vi "ROI entry-Previous ROI compat.vi"(8 "error in (no error)":errorcluster, 11 "Old ROI file path":path) -> (0 "error out":errorcluster, 1 "Proceed":bool, 3 "Old ROI file path (dup)":path, 5 "ROI fit info cluster":T1 {"ROI fit info"."Frame size"."Old" items=["100X100"=100, "128X128"=128, "200X200"=200, "256X256"=256, "512X512"=512, "1024x1024"=1024, "2048x2048"=2048]; "ROI fit info"."Frame size"."New" items=["100X100"=100, "128X128"=128, "200X200"=200, "256X256"=256, "512X512"=512, "1024x1024"=1024, "2048x2048"=2048]})   [LabVIEW 2017]
uses:
  Typedefs/ROI fitting info cluster.ctl
  Typedefs/Frame Size.ctl
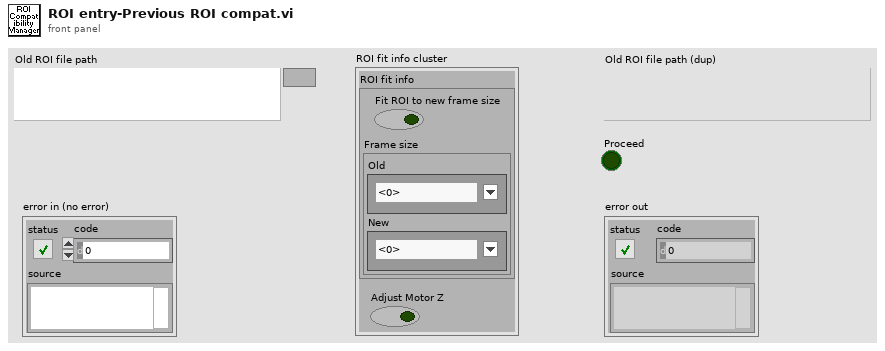
[diagram p1: front panel]
types:
  T1 = typedef "ROI fitting info cluster.ctl" = cluster{"ROI fit info":cluster{"Fit ROI to new frame size":bool, "Frame size":cluster{"Old":T2, "New":T2}}, "Adjust Motor Z":bool}
  T2 = typedef "Frame Size.ctl" = u16
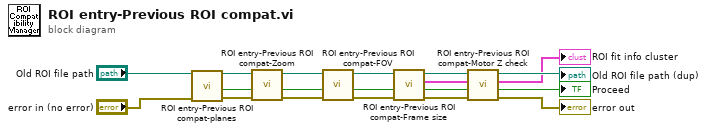
[diagram p0: block diagram]
diagram:
  n1 = call "ROI entry-Previous ROI compat-planes.vi"("error in (no error)"="error in (no error)", "Old ROI file path"="Old ROI file path") -> ("error out"=w17:errorcluster, "Proceed"=w16:bool, "Old ROI file path (dup)"=w15:path)  [unwired: 7 in]
  n2 = call "ROI entry-Previous ROI compat-Zoom.vi"("error in (no error)"=w17, "Proceed"=w16, "Old ROI file path"=w15) -> ("error out"=w6:errorcluster, "Proceed"=w4:bool, "Old ROI file path (dup)"=w2:path)  [unwired: 6 in]
  n3 = call "ROI entry-Previous ROI compat-FOV.vi"("error in (no error)"=w6, "Proceed"=w4, "Old ROI file path"=w2) -> ("error out"=w5:errorcluster, "Proceed"=w3:bool, "Old ROI file path (dup)"=w1:path)  [unwired: 6 in]
  n4 = call "ROI entry-Previous ROI compat-Frame size.vi"("error in (no error)"=w5, "Proceed"=w3, "Old ROI file path"=w1) -> ("error out"=w9:errorcluster, "Proceed"=w8:bool, "ROI fit info"=w7:T1, "Old ROI file path (dup)"=w10:path)  [unwired: 5 in]
  n5 = call "ROI entry-Previous ROI compat-Motor Z check.vi"("error in (no error)"=w9, "Proceed"=w8, "ROI fit info cluster in"=w7, "Old ROI file path"=w10) -> ("error out"=→"error out":errorcluster, "Proceed"=→"Proceed":bool, "ROI fit info cluster"=→"ROI fit info cluster":T1, "Old ROI file path (dup)"=→"Old ROI file path (dup)":path)  [unwired: 4 in]
